vi "Do.vi"(8 "error in (no error)":errorcluster, 10 "Actor in":refnum<class "Actor.lvclass">, 11 "Selftest Device Msg":refnum<class "Selftest Device Msg.lvclass">) -> (0 "error out":errorcluster, 2 "Actor out":refnum<class "Actor.lvclass">)   [LabVIEW 2015, in "CS++DeviceActor.lvlib" / "Selftest Device Msg.lvclass"]
doc: "This VI delivers the message to the actor by calling the appropriate method(s) on the actor."
uses:
  Selftest Device Msg.lvclass
  <vilib>/ActorFramework/Actor/Actor.lvclass
  CS++DeviceActor/CS++DeviceActor.lvclass
  CS++PVMonitor Messages/CS++PVUpdate Msg/CS++PVUpdate Msg.lvclass/CS++PVUpdate Msg.ctl
  Classes/CS++ProcessVariables/ProcessVariable/PV.lvclass/PV.ctl
  Selftest Device Msg.lvclass/Selftest Device Msg.ctl
  Classes/CS++ProcessVariables/ProcessVariable/PV.lvclass
  CS++PVMonitor Messages/CS++PVUpdate Msg/CS++PVUpdate Msg.lvclass
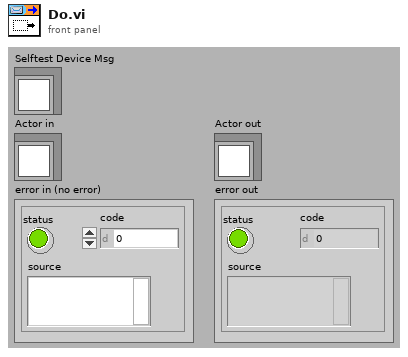
[diagram p1: front panel]
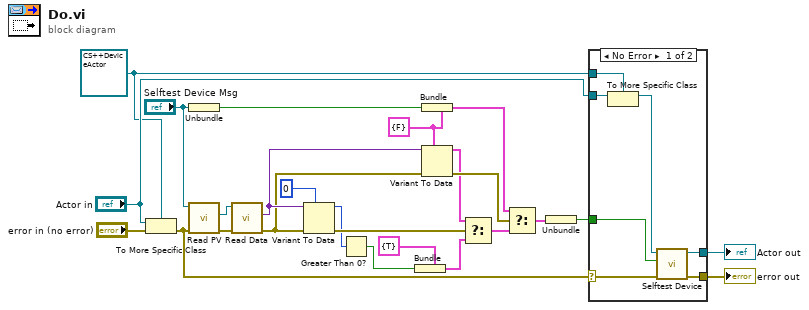
[diagram p0: block diagram]
diagram:
  w17 = cluster{"Self-Test":bool} {"Self-Test"=FALSE} ("Type")
  w21 = refnum<class "CS++DeviceActor.lvclass"> refnum ("Actor in")
  n1 = To More Specific Class(target class=w21, reference="Actor in", error in="error in (no error)") -> (error out=w7:errorcluster)  [unwired: 1 out]
  n2 = Unbundle ("Pre-Unbundler")("Selftest Device Msg") -> (w1:bool)
  n3 = call "Read PV.vi"("error in (no error)"=w7, "CS++PVUpdate Msg in"="Selftest Device Msg") -> ("error out"=w20:errorcluster, "PV"=w16:refnum<class "PV.lvclass">)  [unwired: 7 in, 1 out]
  n4 = call "Read Data.vi"("error in (no error)"=w20, "PV in"=w16) -> ("error out"=w13:errorcluster, "Data"=w14:variant)  [unwired: 7 in, 1 out]
  n5 = Variant To Data ("I16-Conversion")(error in=w13, type=i16 0 ("I16-Conversion-Constant"), Variant=w14) -> (data=w6:i16, error out=w11:errorcluster)
  n6 = Greater Than 0? ("I16-Comp0")(x=w6) -> (x > 0?=w4:bool)
  n7 = Bundle ("I16-Bundle")(cluster=cluster{bool} {TRUE} ("I16-Cluster"), w4) -> (w3:cluster{bool})
  n8 = Bundle ("Pre-Bundler")(cluster=w17, "Self-Test"=w1) -> (w18:cluster{"Self-Test":bool})
  n9 = Variant To Data(error in=w13, type=w17, Variant=w14) -> (data=w10:cluster{"Self-Test":bool}, error out=w19:errorcluster)
  n10 = Select ("I16-Select")(t=w10, s=w11, f=w3) -> (s? t:f=w9:cluster{"Self-Test":bool})
  n11 = Select ("MainSelect")(t=w18, s=w19, f=w9) -> (s? t:f=w12:cluster{"Self-Test":bool})
  n12 = Unbundle ("Main-Unbundler")(w12) -> ("Self-Test"=w2:bool)
  n13 = case shown="No Error" w7 {
    selector: w7 -> [w30 w34]
    tunnel: [w32 w34] -> w24
    tunnel: [w31 w33] -> w23
    tunnel: "Actor in" -> [w29 w33]
    tunnel: w21 -> [w28 _]
    tunnel: w2 -> [w26 _]
    frame No Error {
      n14 = To More Specific Class(target class=w28, reference=w29) -> (specific class reference=w27:refnum<class "CS++DeviceActor.lvclass">)  [unwired: 1 in, 1 out]
      n15 = call "Selftest Device.vi"("error in (no error)"=w30, "Self-Test"=w26, "CS++DeviceActor in"=w27) -> ("error out"=w32:errorcluster, "CS++DeviceActor out"=w31:refnum<class "CS++DeviceActor.lvclass">)  [unwired: 7 in]
    }
    frame Error {
    }
  }
  "error out" <- w24
  "Actor out" <- w23
